vi "GetExampleImage.vi"(8 "error in":errorcluster, 11 "File Path":path) -> (0 "error out":errorcluster, 3 "path":path)   [LabVIEW 2020, in "OpenLvVision_Image.lvlib"]
uses:
  OpenLvVision_Image.lvlib
  <vilib>/registry/registry.llb/Registry SAM.ctl
  <vilib>/registry/registry.llb/Read Registry Value Simple STR.vi
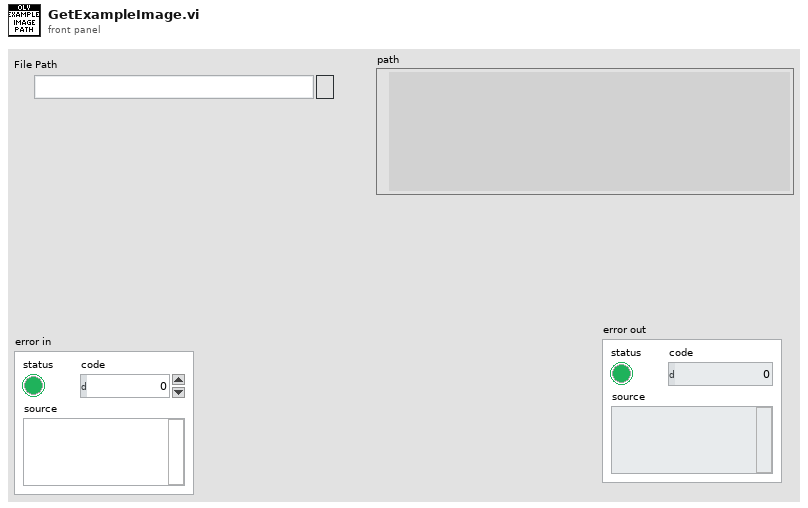
[diagram p1: front panel]
types:
  T1 = typedef "Registry SAM.ctl" = enum32{"KEY_QUERY_VALUE", "KEY_SET_VALUE", "KEY_CREATE_SUB_KEY", "KEY_ENUMERATE_SUB_KEYS", "KEY_NOTIFY", "KEY_CREATE_LINK", "KEY_READ", "KEY_WRITE", "KEY_ALL_ACCESS", "KEY_READ | KEY_WRITE"}
  T2 = typedef "Registry refnum.ctl" = refnum<k1>
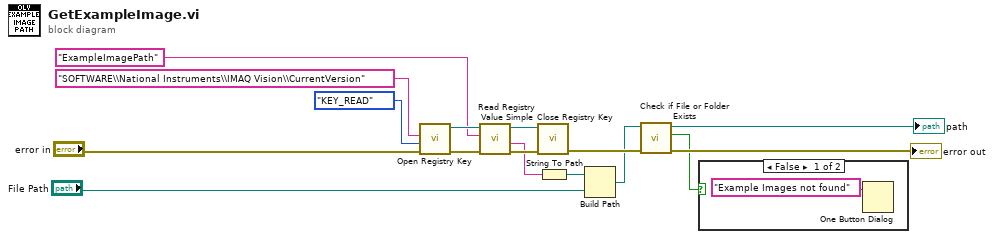
[diagram p0: block diagram]
diagram:
  n1 = call <vilib>:"Open Registry Key.vi"("error in (no error)"="error in", "security access mask (KEY_READ | KEY_WRITE)"=Registry_SAM."KEY_READ", "subkey"="SOFTWARE\\National Instruments\\IMAQ Vision\\CurrentVersion") -> ("error out"=w15:errorcluster, "refnum out"=w14:T2)  [unwired: 7 in]
  n2 = call-poly <vilib>:"Read Registry Value Simple.vi"("error in (no error)"=w15, "value"="ExampleImagePath", "refnum"=w14) -> ("error out"=w12:errorcluster, "String/Binary data"=w10:string, "refnum out"=w11:T2)  [unwired: 3 in, 1 out]
  n3 = call <vilib>:"Close Registry Key.vi"("error in (no error)"=w12, "refnum"=w11) -> ("error out"=w5:errorcluster)  [unwired: 5 in]
  n4 = String To Path(string=w10) -> (path=w8:path)
  n5 = Build Path(base path=w8, name or relative path="File Path") -> (appended path=w3:path)
  n6 = call <vilib>:"Check if File or Folder Exists.vi"("error in (no error)"=w5, "path"=w3) -> ("error out"=→"error out":errorcluster, "file or folder exists?"=w1:bool, "dup path"=→"path":path)  [unwired: 7 in]
  n7 = case shown="False" w1 {
    frame False {
      n8 = One Button Dialog(message="Example Images not found") -> ()  [unwired: 1 in, 1 out]
    }
    frame True {
    }
  }
